vi "Kinematics.vi"() -> ()   [LabVIEW 2021]
uses:
  <vilib>/express/express arith-compare/Formula/XNode/ExpressFormulaBlockNode.xnode
panel:
  in  "?":bool
  in  "?":bool
  in  "?":bool
  in  "Mass":dbl min=0.0
  in  "Velocity":dbl=10.0 min=0.0
  in  "Angle":dbl=45.0 min=-0.0 max=89.0
  in  "Height (Initial)":dbl=10.0 min=0.0
  out "Trajectory Plot":cluster{dbl[], dbl[]}[](graph)
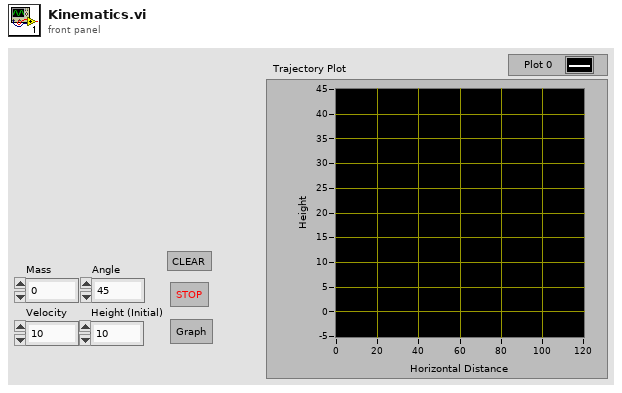
[diagram p1: front panel]
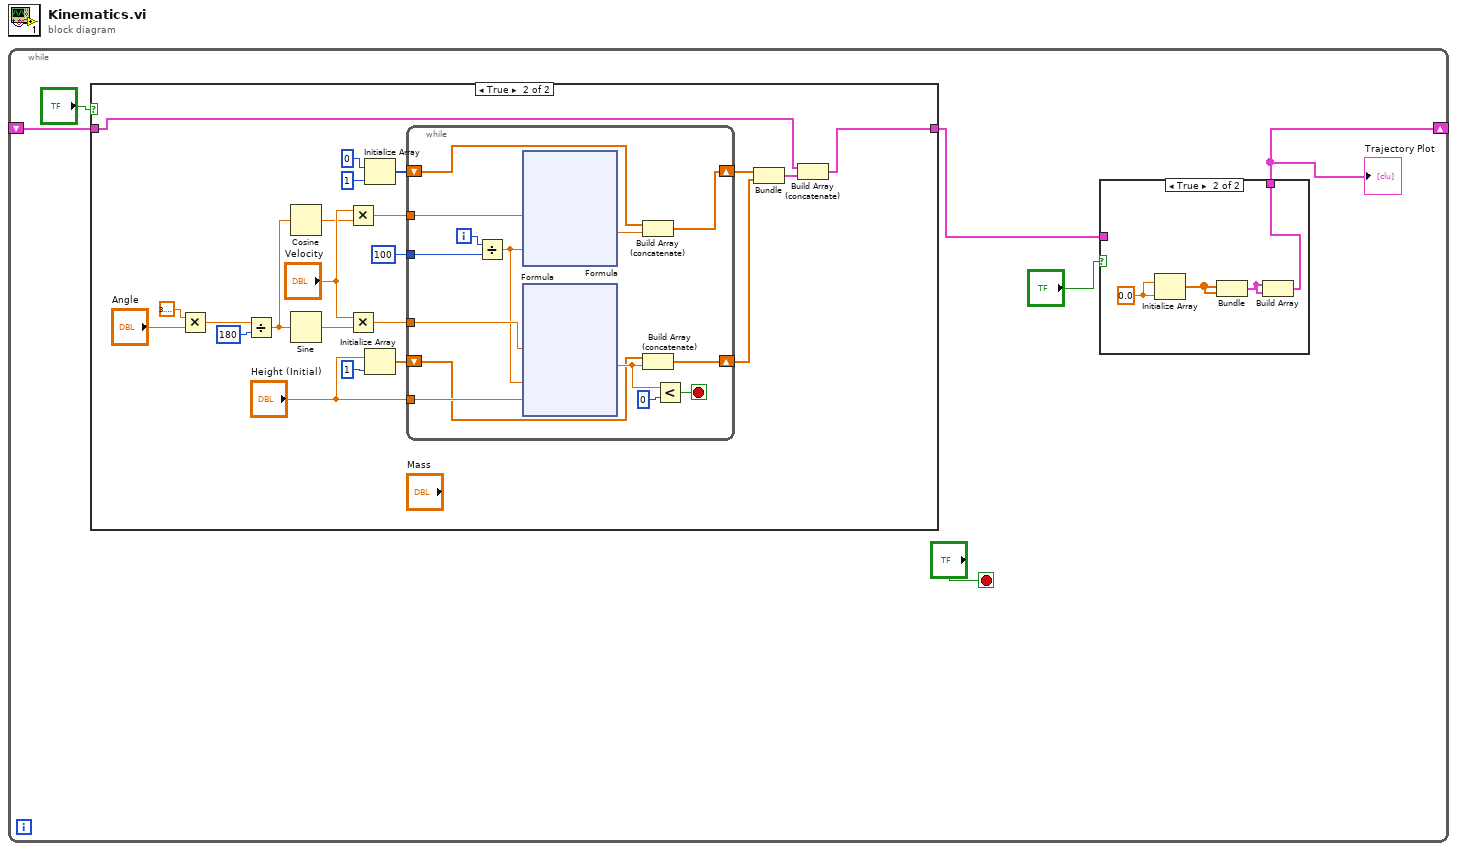
[diagram p0: block diagram]
diagram:
  n1 = while {
    shift-right: [w1] -> _
    shift-left: _ -> [w6]
    stop <- "?" stop-if-true
    n2 = case shown="True" "?" {
      tunnel: w6 -> [w12 w21]
      tunnel: [w12 w20] -> w2
      frame False {
      }
      frame True {
        n3 = Multiply(x=3.141592653589793, y="Angle") -> (x*y=w32:dbl)
        n4 = Divide(x=w32, y=180) -> (x/y=w30:dbl)
        n5 = Cosine(x=w30) -> (cos(x)=w26:dbl)
        n6 = Sine(x=w30) -> (sin(x)=w29:dbl)
        n7 = Multiply(x="Velocity", y=w26) -> (x*y=w25:dbl)
        n8 = Multiply(x="Velocity", y=w29) -> (x*y=w28:dbl)
        n9 = Initialize Array(0, 1) -> (w14:i32[])
        n10 = Initialize Array("Height (Initial)", 1) -> (w17:dbl[])
        n11 = while {
          tunnel: w28 -> [w45]
          tunnel: w25 -> [w46]
          tunnel: "Height (Initial)" -> [w43]
          tunnel: 100 -> [w47]
          shift-right: [w37] -> w23
          shift-left: w17 -> [w35]
          shift-right: [w38] -> w24
          shift-left: w14 -> [w36]
          i -> [w48]
          stop <- w41 stop-if-true
          n12 = Divide(x=w48, y=w47) -> (x/y=w44:dbl)
          n13 = xnode "Formula"("V_X"=w46, "T"=w44) -> ("Result"=w39:dbl)  [unwired: 1 in, 1 out]
          n14 = xnode "Formula"("V_Y"=w45, "T"=w44, "Y_I"=w43) -> ("Result"=w40:dbl)  [unwired: 1 in, 1 out]
          n15 = Build Array (concatenate)(w36, w39) -> (w38:dbl[])
          n16 = Build Array (concatenate)(w35, w40) -> (w37:dbl[])
          n17 = Less?(x=w40, y=0) -> (x < y?=w41:bool)
        }
        n18 = Bundle(w24, w23) -> (w22:cluster{dbl[], dbl[]})  [unwired: 1 in]
        n19 = Build Array (concatenate)(w21, w22) -> (w20:cluster{dbl[], dbl[]}[])
      }
    }
    n20 = case shown="True" "?" {
      tunnel: [w7 w8] -> w1
      tunnel: w2 -> [w7 _]
      frame False {
      }
      frame True {
        w11 = 0.0
        n21 = Initialize Array(w11, w11) -> (w10:dbl[])
        n22 = Bundle(w10, w10) -> (w9:cluster{dbl[], dbl[]})  [unwired: 1 in]
        n23 = Build Array(w9, w9) -> (w8:cluster{dbl[], dbl[]}[])
      }
    }
    "Trajectory Plot" <- w1
  }
